vi "Device Launcher - Wait For Startup.vi"(0 "Notifier Name":string, 11 "Wait Time (ms)":i32) -> (4 "Notifier Name (Dup)":string, 15 "Running?":bool)   [LabVIEW 2016]
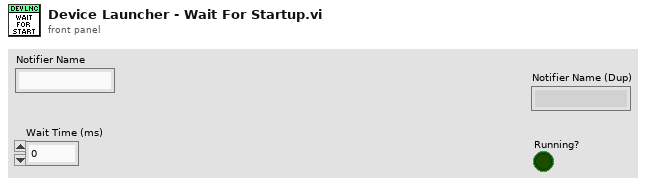
[diagram p1: front panel]
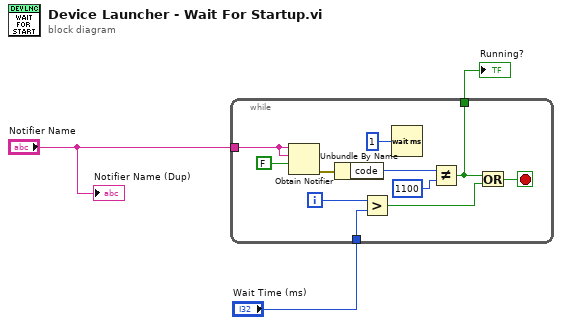
[diagram p0: block diagram]
diagram:
  n1 = while {
    tunnel: "Notifier Name" -> [w14]
    tunnel: [w5] -> w2
    tunnel: "Wait Time (ms)" -> [w4]
    i -> [w11]
    stop <- w6 stop-if-true
    n2 = Obtain Notifier(name (unnamed)=w14, notification data type=w14, create if not found? (T)=FALSE) -> (error out=w12:errorcluster)  [unwired: 1 in, 2 out]
    n3 = Unbundle By Name(w12) -> ("code"=w10:i32)
    n4 = Greater?(x=w11, y=w4) -> (0:w7:bool)
    n5 = Wait (ms)(milliseconds to wait=u32 1) -> ()  [unwired: 1 out]
    n6 = Not Equal?(x=w10, y=1100) -> (x != y?=w5:bool)
    n7 = Or(x=w5, y=w7) -> (x .or. y?=w6:bool)
  }
  "Running?" <- w2
  "Notifier Name (Dup)" <- "Notifier Name"
